vi "Rearrange Instr.vi"(6 "Item to Move":i32, 7 "Insert At":i32, 8 "Configured Names":string[](array[string]), 9 "Setup In":T1[](array[typedef]) {"Private"."Offset" format="%^_3e"; "Private"."Scale Factors" format="%^_3e"}) -> (1 "NewVal Out":i32, 2 "Item Names":string[](array[string]), 3 "Setup Out":T1[](array[typedef]) {"Private"."Offset" format="%^_3e"; "Private"."Scale Factors" format="%^_3e"})   [LabVIEW 2020]
uses:
  Sub Controls/Instrument Properties.ctl
  Sub Controls/Public.ctl
  Sub Controls/Private.ctl
  Sub Controls/Instrument Ref.ctl
  Sub Controls/SystemCheckBox-resize.ctl
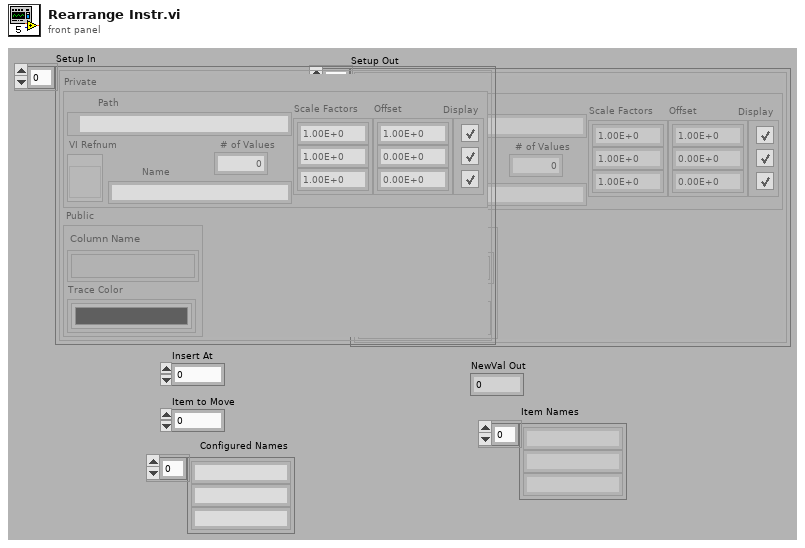
[diagram p1: front panel]
types:
  T1 = typedef "Instrument Properties.ctl" = cluster{"Public":T2, "Private":T3}
  T2 = typedef "Public.ctl" = cluster{"Column Name":string[], "Trace Color":u32[]}
  T3 = typedef "Private.ctl" = cluster{"Path":path, "VI Refnum":T4, "Name":string, "# of Values":i32, "Scale Factors":dbl[], "Display":T5[], "Offset":dbl[]}
  T4 = typedef "Instrument Ref.ctl" = refnum<vi>
  T5 = typedef "SystemCheckBox-resize.ctl" = bool
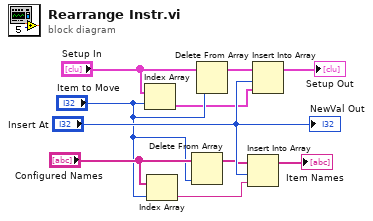
[diagram p0: block diagram]
diagram:
  n1 = Index Array(array="Setup In", index="Item to Move") -> (element=w3:T1)
  n2 = Index Array(array="Configured Names", index="Item to Move") -> (element=w1:string)
  n3 = Delete From Array(array="Configured Names", index="Item to Move") -> (array with subset deleted=w2:string[])  [unwired: 1 in, 1 out]
  n4 = Delete From Array(array="Setup In", index="Item to Move") -> (array with subset deleted=w4:T1[])  [unwired: 1 in, 1 out]
  n5 = Insert Into Array(array=w2, index="Insert At", new element=w1) -> (→"Item Names":string[])
  n6 = Insert Into Array(array=w4, index="Insert At", new element=w3) -> (→"Setup Out":T1[])
  "NewVal Out" <- "Insert At"
